vi "Prepare Log.vi"(8 "error in (no error)":errorcluster, 10 "Prepare Log":T1, 11 "Data Logger Module in":refnum<class "Data Logger DBL Module.lvclass">) -> (0 "error out":errorcluster, 3 "Data Logger Module out":refnum<class "Data Logger DBL Module.lvclass">)   [LabVIEW 2020, in "VolatusData.lvlib" / "Data Logger DBL Module.lvclass"]
uses:
  Data Logger DBL Module.lvclass
  C:/dev/lv20CE/relink/lv-volatus/Volatus/Module/Module.lvclass
  Prepare Log.ctl
  Data Logger DBL Module.lvclass/Data Logger DBL Module.ctl
  Volatus/Module/Module.lvclass/Module.ctl
  Logger Ready.ctl
  Volatus/MessageQ/MessageQ.lvclass/MessageQ.ctl
  Volatus/Module/Parent Q.vi
  Volatus/MessageQ/MessageQ.lvclass
  VolatusData.lvlib
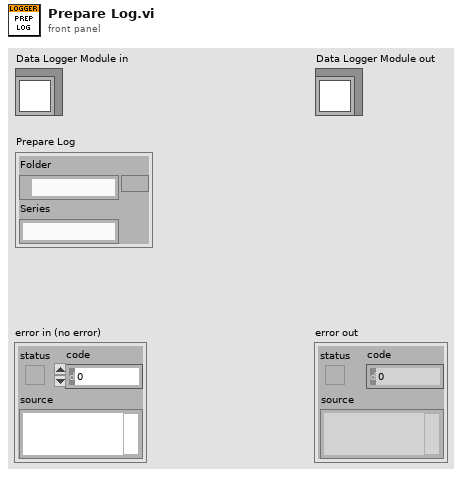
[diagram p1: front panel]
types:
  T1 = typedef "VolatusData.lvlib/Prepare Log.ctl" = cluster{"Folder":path, "Series":string}
  T2 = enum16{"open", "open or create", "create or replace", "create", "open (read-only)"}
  T3 = typedef "VolatusData.lvlib/Logger Ready.ctl" = cluster{"ID":string}
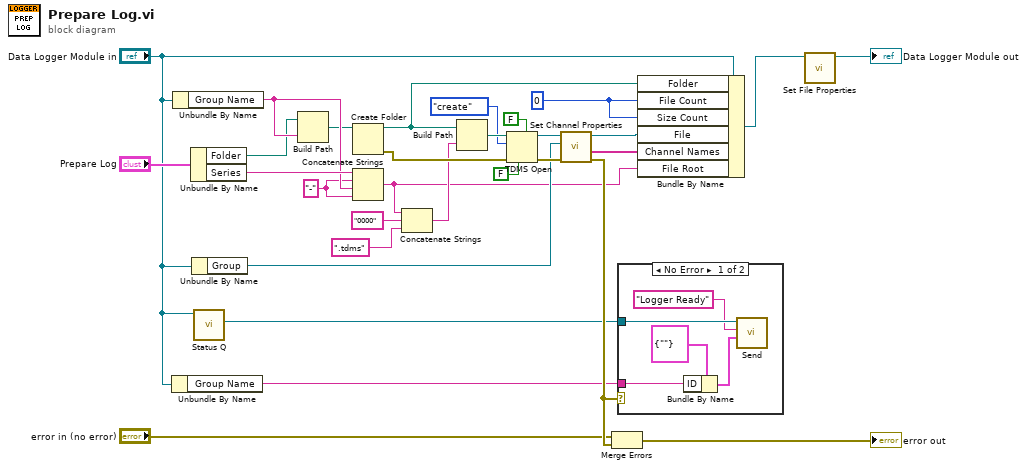
[diagram p0: block diagram]
diagram:
  w20 = 0
  w22 = "-" ("string")
  n1 = Unbundle By Name("Data Logger Module in") -> ("Group Name"=w1:string)
  n2 = Unbundle By Name("Data Logger Module in") -> ("Group Name"=w24:string)
  n3 = Unbundle By Name("Prepare Log") -> ("Folder"=w7:path, "Series"=w25:string)
  n4 = Unbundle By Name("Data Logger Module in") -> ("Group"=w13:refnum<class "Group DBL.lvclass">)
  n5 = call "Status Q.vi"("Data Logger Module in"="Data Logger Module in") -> ("Status Q"=w3:refnum<class "MessageQ.lvclass">)  [unwired: 9 in, 1 out]
  n6 = Build Path(base path=w7, name or relative path=w24) -> (appended path=w23:path)
  n7 = Create Folder(path (use dialog)=w23) -> (created path=w4:path, error out=w28:errorcluster)  [unwired: 2 in, 1 out]
  n8 = Concatenate Strings(w25, w22, w24, w22) -> (w6:string)
  n9 = Concatenate Strings(w6, "0000" ("string"), ".tdms" ("string")) -> (w8:string)
  n10 = Build Path(base path=w4, name or relative path=w8) -> (appended path=w18:path)
  n11 = TDMS Open(5:FALSE ("create index file? (T)"), 6:FALSE ("disable buffering? (T)"), 8:w28, 10:T2."create" ("operation (0:open)"), 11:w18) -> (0:w29:errorcluster, 3:w14:refnum<k34>)  [unwired: 2 in]
  n12 = call "Set Channel Properties.vi"("error in (no error)"=w29, "Group"=w13, "File in"=w14) -> ("error out"=w30:errorcluster, "Channel Names"=w11:string[], "File"=w12:refnum<k34>)  [unwired: 5 in, 1 out]
  n13 = Merge Errors("error in (no error)", w30) -> (→"error out":errorcluster)
  n14 = case shown="No Error" w30 {
    tunnel: w3 -> [w35 _]
    tunnel: w1 -> [w31 _]
    frame No Error {
      n15 = Bundle By Name(cluster=T3 {"ID"=""} ("Logger Ready"), "ID"=w31) -> (w33:T3)
      n16 = call "Send.vi"("Data"=w33, "ID"="Logger Ready", "MessageQ in"=w35) -> ()  [unwired: 7 in, 2 out]
    }
    frame Error {
    }
  }
  n17 = Bundle By Name(cluster="Data Logger Module in", "Folder"=w4, "File Count"=w20, "Size Count"=w20, "File"=w12, "Channel Names"=w11, "File Root"=w6) -> (w21:refnum<class "Data Logger DBL Module.lvclass">)
  n18 = call "Set File Properties.vi"("Data Logger Module in"=w21) -> ("Data Logger Module out"=→"Data Logger Module out":refnum<class "Data Logger DBL Module.lvclass">)  [unwired: 9 in, 1 out]
